vi "LoopScript_ChangeRadiusManyRuns.vi"() -> ()   [LabVIEW 2017]
uses:
  FrontPanelReferences.vi
  ImageAcquisitionProgram/ImageAcquisitionLibrary/GlobalFrontPanelReferences.vi
  AODExperimentControls/AODControl/AODGlobals.vi
  AODControl/MessageQueue/QueueOperations/Enqueue Message (Single).vi
  WaveformGenerator.lvlib
  ImageAcquisitionProgram/ImageAcquisitionLibrary/ImageAcquisitionLibrary.lvlib
  AODControl/AODControl.lvlib
  AODControl/MessageQueue/MessageQueue.lvlib
panel:
  out "Started":bool=TRUE
  out "Radius":dbl[](array[numeric])
  in  "Run":bool
  in  "No Of Points":i32=21
  in  "Stop Between fwd/bwd":bool
  out "Current Radius":dbl=3.48
  in  "R_f":dbl=3.38
  in  "R_0":dbl=3.5
  in  "Radius Steps":i32=6
  out "Current Step Down":i32=199
  out "Current Step Up":i32=180
  out "Current Loop":i32
  in  "NumberOfLoops":i32=100
  in  "Record Time":u32=1000
  in  "B_f^2":dbl=1.0
  in  "B_0^2":dbl
  in  "Torque Steps":i32=200
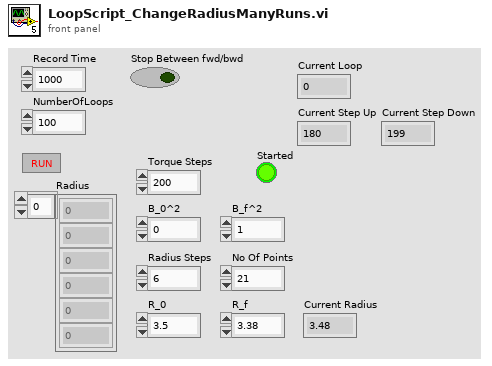
[diagram p1: front panel]
types:
  T1 = typedef "AODControl.lvlib/MessageQueue.lvlib/All Message Queues.ctl" = cluster{" AOD Interface":refnum<queue>}
  T2 = typedef "ImageAcquisitionLibrary.lvlib/References.ctl" = cluster{"Acquire":refnum<vi>, "Rec":refnum<vi>, "Tracking":refnum<vi>, "Settings":refnum<vi>, "Stop":refnum<vi>, "Initialized?":bool, "ImDisplay":refnum<vi>}
  T3 = typedef "WaveformGenerator.lvlib/WaveformGeneratorInterfaceRef.ctl" = cluster{"Waveform X":refnum<vi>, "Waveform Y":refnum<vi>, "Waveform Z":refnum<vi>, "Amplitude X":refnum<vi>, "Amplitude Y":refnum<vi>, "Amplitude Z":refnum<vi>, "Frequency X":refnum<vi>, "Frequency Y":refnum<vi>, "Frequency Z":refnum<vi>, "Phase X":refnum<vi>, "Phase Y":refnum<vi>, "Phase Z":refnum<vi>, "Offset X":refnum<vi>, "Offset Y":refnum<vi>, "Offset Z":refnum<vi>, "Stop":refnum<vi>, "On/Off":refnum<vi>, "Field^2":refnum<vi>}
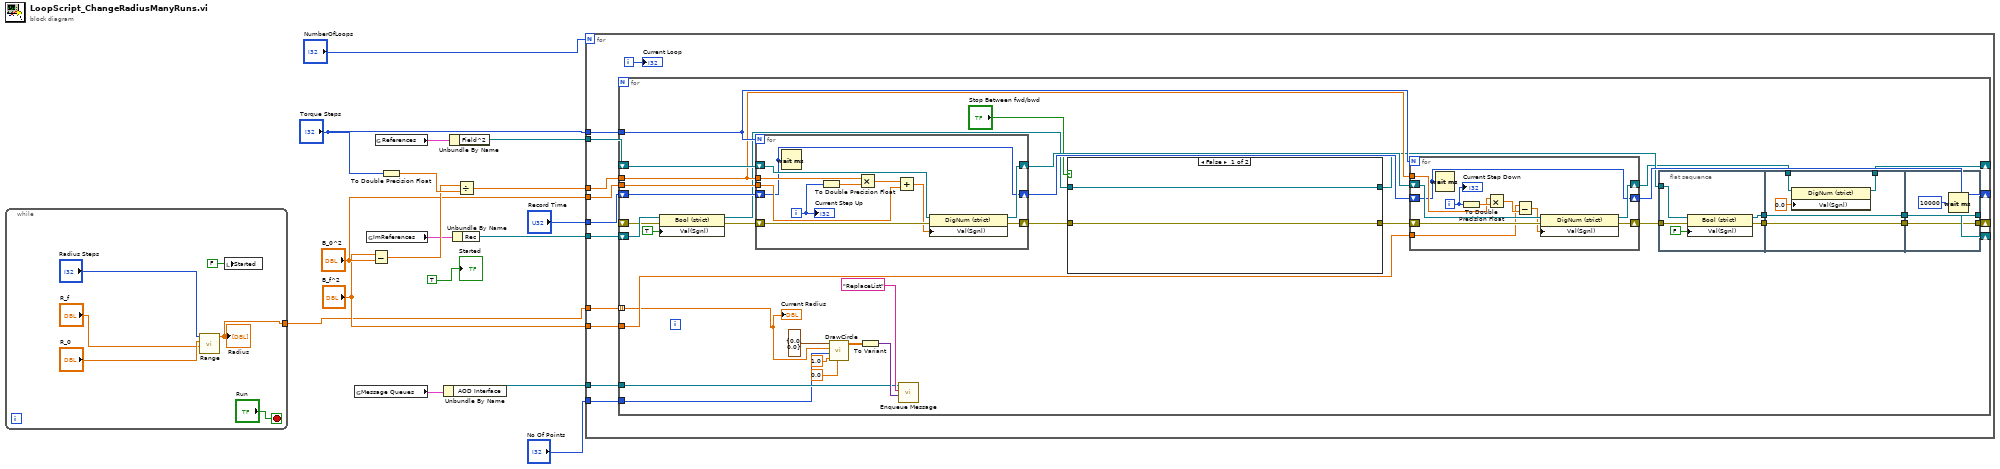
[diagram p0: block diagram]
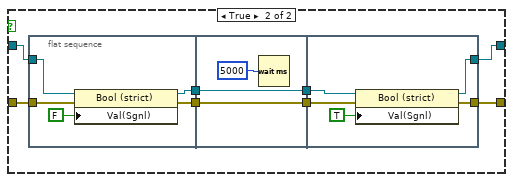
[diagram p2: hidden frame]
diagram:
  n1 = while {
    tunnel: [w20] -> w2
    stop <- "Run" stop-if-true
    n2 = call "Range.vi"("End"="R_f", "Start"="R_0", "Steps"="Radius Steps") -> ("Array"=w20:dbl[])  [unwired: 8 in]
    "Radius" <- w20
    n3 = local write "Started"(FALSE ("Waiting")) -> ()
  }
  n4 = global read "AODGlobals.vi" "Message Queues"() -> (w6:T1)
  n5 = global read "GlobalFrontPanelReferences.vi" "ImReferences"() -> (w8:T2)
  n6 = Subtract(x="B_f^2", y="B_0^2") -> (x-y=w14:dbl)
  n7 = global read "FrontPanelReferences.vi" "References"() -> (w17:T3)
  n8 = To Double Precision Float(number="Torque Steps") -> (double precision float=w15:dbl)
  n9 = Unbundle By Name(w6) -> ("AOD Interface"=w5:refnum<queue>)
  n10 = Unbundle By Name(w17) -> ("Field^2"=w16:refnum<vi>)
  n11 = Unbundle By Name(w8) -> ("Rec"=w7:refnum<vi>)
  n12 = Divide(x=w14, y=w15) -> (x/y=w11:dbl)
  n13 = for {
    N: "NumberOfLoops" -> [_]
    tunnel: w16 -> [w34]
    tunnel: "Record Time" -> [w33]
    tunnel: "Torque Steps" -> [w32]
    tunnel: w11 -> [w31]
    tunnel: "B_0^2" -> [w30]
    tunnel: "B_f^2" -> [w29]
    tunnel: w7 -> [w28]
    tunnel: w5 -> [w27]
    tunnel: "No Of Points" -> [w25]
    tunnel: w2 -> [w24]
    i -> [w26]
    n14 = for {
      tunnel: w32 -> [w68]
      tunnel: w31 -> [w65]
      tunnel: w30 -> [w64]
      shift-right: [w51] -> _
      shift-left: _ -> [w55]
      shift-right: [w35] -> _
      shift-left: w34 -> [w70]
      shift-right: [w63] -> _
      shift-left: w33 -> [w69]
      tunnel: w29 -> [w62]
      shift-right: [w53] -> _
      shift-left: w28 -> [w56]
      tunnel: w27 -> [w43]
      tunnel: w25 -> [w42]
      tunnel: w24 -> [w41] mode=indexing
      n15 = property class="Bool (strict)"(reference=w56, error in=w55, "Val(Sgnl)"=TRUE ("Value (Signaling)")) -> (reference out=w58:refnum<vi>, error out=w59:errorcluster)
      n16 = for {
        N: w68 -> [_]
        shift-right: [w121] -> w66
        shift-left: w70 -> [w128]
        shift-right: [w120] -> w61
        shift-left: w59 -> [w127]
        tunnel: w64 -> [w126]
        tunnel: w65 -> [w124]
        shift-right: [w119] -> w67
        shift-left: w69 -> [w119]
        i -> [w118]
        n17 = Wait (ms)(milliseconds to wait=w119) -> ()  [unwired: 1 out]
        n18 = To Double Precision Float(number=w118) -> (double precision float=w125:dbl)
        n19 = Multiply(x=w124, y=w125) -> (x*y=w123:dbl)
        n20 = Add(x=w123, y=w126) -> (x+y=w122:dbl)
        n21 = property class="DigNum (strict)"(reference=w128, error in=w127, "Val(Sgnl)"=w122) -> (reference out=w121:refnum<vi>, error out=w120:errorcluster)
        "Current Step Up" <- w118
      }
      n22 = call "DrawCircle.vi"("Phase"=0.0, "Eccentricity"=1.0, "No Of Points"=w42, "Radius"=w41, "Center"=cluster{"X":dbl, "Y":dbl} {"X"=0.0, "Y"=0.0}) -> ("Array"=w45:dbl[][])  [unwired: 6 in]
      n23 = To Variant(anything=w45) -> (Variant=w44:variant)
      n24 = call-poly "Enqueue Message.vi"("Message Data"=w44, "Message"="ReplaceList", "Message Queue"=w43) -> ()  [unwired: 7 in, 2 out]
      n25 = case shown="False" "Stop Between fwd/bwd" {
        tunnel: w61 -> [w71 w76]
        tunnel: [w71 w75] -> w60
        tunnel: w58 -> [w72 w74]
        tunnel: [w72 w73] -> w54
        frame False {
        }
        frame True {
          n26 = flat-sequence {
            tunnel: w76 -> [w85]
            tunnel: w74 -> [w84]
            tunnel: [w82] -> w80
            tunnel: [w81] -> w79
            tunnel: [w87] -> w78
            tunnel: w80 -> [w87]
            tunnel: [w86] -> w77
            tunnel: w79 -> [w86]
            tunnel: w78 -> [w93]
            tunnel: w77 -> [w92]
            tunnel: [w90] -> w73
            tunnel: [w89] -> w75
            frame #0 {
              n27 = property class="Bool (strict)"(reference=w84, error in=w85, "Val(Sgnl)"=FALSE ("Value (Signaling)")) -> (reference out=w82:refnum<vi>, error out=w81:errorcluster)
            }
            frame #1 {
              n28 = Wait (ms)(milliseconds to wait=u32 5000) -> ()  [unwired: 1 out]
            }
            frame #2 {
              n29 = property class="Bool (strict)"(reference=w93, error in=w92, "Val(Sgnl)"=TRUE ("Value (Signaling)")) -> (reference out=w90:refnum<vi>, error out=w89:errorcluster)
            }
          }
        }
      }
      n30 = for {
        N: w68 -> [_]
        shift-right: [w113] -> w36
        shift-left: w66 -> [w117]
        shift-right: [w112] -> w52
        shift-left: w60 -> [w116]
        tunnel: w62 -> [w107]
        tunnel: w65 -> [w114]
        shift-right: [w111] -> w63
        shift-left: w67 -> [w111]
        i -> [w109]
        n31 = Wait (ms)(milliseconds to wait=w111) -> ()  [unwired: 1 out]
        n32 = To Double Precision Float(number=w109) -> (double precision float=w115:dbl)
        n33 = Multiply(x=w114, y=w115) -> (x*y=w108:dbl)
        n34 = Subtract(x=w107, y=w108) -> (x-y=w110:dbl)
        n35 = property class="DigNum (strict)"(reference=w117, error in=w116, "Val(Sgnl)"=w110) -> (reference out=w113:refnum<vi>, error out=w112:errorcluster)
        "Current Step Down" <- w109
      }
      n36 = flat-sequence {
        tunnel: w52 -> [w98]
        tunnel: w54 -> [w97]
        tunnel: [w95] -> w40
        tunnel: [w94] -> w38
        tunnel: w40 -> [w103]
        tunnel: [w103] -> w39
        tunnel: w38 -> [w102]
        tunnel: [w102] -> w37
        tunnel: w36 -> [w101]
        tunnel: [w100] -> w35
        tunnel: w39 -> [w105]
        tunnel: w37 -> [w104]
        tunnel: [w105] -> w53
        tunnel: [w104] -> w51
        frame #0 {
          n37 = property class="Bool (strict)"(reference=w97, error in=w98, "Val(Sgnl)"=FALSE ("Value (Signaling)")) -> (reference out=w95:refnum<vi>, error out=w94:errorcluster)
        }
        frame #1 {
          n38 = property class="DigNum (strict)"(reference=w101, "Val(Sgnl)"=0.0 ("Value (Signaling)")) -> (reference out=w100:refnum<vi>)  [unwired: 1 in, 1 out]
        }
        frame #2 {
          n39 = Wait (ms)(milliseconds to wait=u32 10000) -> ()  [unwired: 1 out]
        }
      }
      "Current Radius" <- w41
    }
    "Current Loop" <- w26
  }
  "Started" <- TRUE ("Boolean")
